vi "instrument_close.vi"(8 "pld_3605_error_input":errorcluster, 9 "pld_3605":refnum<visa-resource-name>, 10 "keithley_6510_error_input":errorcluster, 11 "keithley_6510":refnum<visa-resource-name>) -> ()   [LabVIEW 2019]
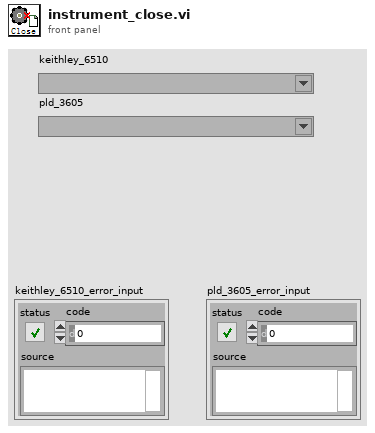
[diagram p1: front panel]
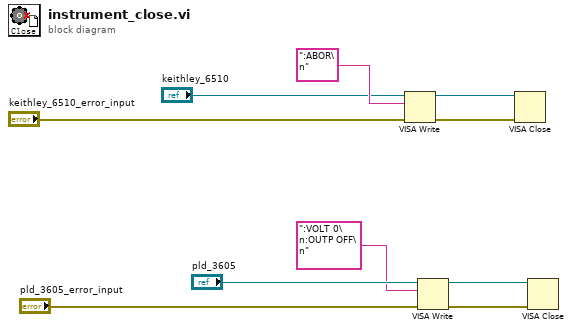
[diagram p0: block diagram]
diagram:
  n1 = VISA Write(VISA resource name="keithley_6510", write buffer=":ABOR\n", error in (no error)="keithley_6510_error_input") -> (VISA resource name out=w10:refnum<visa-resource-name>, error out=w9:errorcluster)  [unwired: 1 out]
  n2 = VISA Write(VISA resource name="pld_3605", write buffer=":VOLT 0\n:OUTP OFF\n", error in (no error)="pld_3605_error_input") -> (VISA resource name out=w4:refnum<visa-resource-name>, error out=w5:errorcluster)  [unwired: 1 out]
  n3 = VISA Close(VISA resource name=w10, error in (no error)=w9) -> ()  [unwired: 1 out]
  n4 = VISA Close(VISA resource name=w4, error in (no error)=w5) -> ()  [unwired: 1 out]
